vi "list tdms files.vi"(0 "reference in":refnum<class "TDMS_DataHandler.lvclass">, 5 "error in (no error)":errorcluster) -> (14 "reference out":refnum<class "TDMS_DataHandler.lvclass">, 16 "tdms file paths":path[](array[path]), 19 "error out":errorcluster)   [LabVIEW 2019, in "TDMS_DataHandler.lvclass"]
doc: "Get all tdms files from file directory"
uses:
  TDMS_DataHandler.lvclass
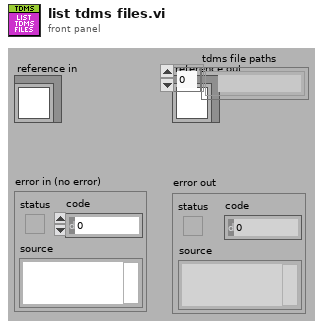
[diagram p1: front panel]
types:
  T1 = typedef "TDMS_DataHandler.lvclass/ObjectAttributes.ctl" = cluster{"Directory":path, "FilePath":path, "FileRef":refnum<k34>, "ExperimentName":string, "GroupName":string, "ChannelNames":string[], "Datum":waveform(dbl)[], "Group_Metadata":cluster{"property names":string[], "property values":variant[]}, "Channel_Metadata":cluster{"property names":string[], "property values":variant[]}}
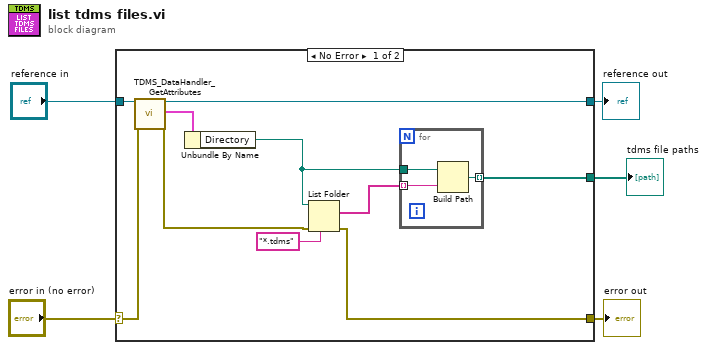
[diagram p0: block diagram]
diagram:
  n1 = case shown="No Error" "error in (no error)" {
    selector: "error in (no error)" -> [w15 w20]
    tunnel: [w9 w20] -> w4
    tunnel: [w14 w19] -> w2
    tunnel: "reference in" -> [w12 w19]
    tunnel: [w6 _] -> w1
    frame No Error {
      n2 = call "TDMS_DataHandler_GetAttributes.vi"("reference in"=w12, "error in (no error)"=w15) -> ("reference out"=w14:refnum<class "TDMS_DataHandler.lvclass">, "attributes"=w13:T1, "error out"=w10:errorcluster)  [unwired: 14 in, 1 out]
      n3 = Unbundle By Name(w13) -> ("Directory"=w8:path)
      n4 = List Folder(path=w8, pattern="*.tdms", error in=w10) -> (filenames=w7:string[], error out=w9:errorcluster)  [unwired: 1 in, 2 out]
      n5 = for {
        tunnel: w8 -> [w18]
        tunnel: w7 -> [w17] mode=indexing
        tunnel: [w16] -> w6 mode=indexing
        n6 = Build Path(base path=w18, name or relative path=w17) -> (appended path=w16:path)
      }
    }
    frame Error {
    }
  }
  "error out" <- w4
  "reference out" <- w2
  "tdms file paths" <- w1
